vi "Mono Test App.vi"() -> ()   [LabVIEW 2009]
panel:
  in  "BtnCurrent Grating":bool
  out "Current Grating":dbl
  in  "Grating Index":i32
  out "Grating array":dbl[](array[numeric])
  in  "Available Gratings":bool
  in  "Turret Control":bool
  in  "Actual Wavlength":dbl caption="Enter Actual Wavlength"
  in  "Calibrate":bool
  out "Current WL":dbl
  in  "Target WL":dbl
  in  "Get Cur WL":bool
  in  "Move to WL":bool
  in  "Mirror Position  2":u16(ring) caption="Target Position" items=["Front", "Side"]
  in  "Slit Width External":dbl caption="Target Slit Width"
  in  "Slit External":u16(ring) caption="Slit" items=["Front Entrance", "Side Entrance", "Front Exit", "Side Exit", "First Intermediate", "Second Intermediate"]
  out "Slit Width":dbl caption="Current Slit Width"
  in  "Slit":u16(ring) items=["Front Entrance", "Side Entrance", "Front Exit", "Side Exit", "First Intermediate", "Second Intermediate"]
  in  "Set Slit":bool
  in  "Get Slit":bool
  in  "Mirror Number   2":u16(ring) caption="Mirror Number" items=["Entrance", "Exit"]
  in  "Set Mirror Pos":bool
  in  "Get Mirror Pos":bool
  out "Mirror Position":i32(ring) caption="Current  Position" items=["EntranceMirror", "ExitMirror", "Front", "Side"]
  in  "Mirror Number":u16(ring) items=["Entrance", "Exit"]
  in  "stop":bool
  in  "MonoRefNum":refnum<k7>
  out "Initialized":bool
  in  "Force Init":bool
  in  "UniqueID":string
  in  "error in (no error)":errorcluster
  # "Force Init"
  # "Don't Force"
  # "Indexes in this array are zero based"
  # "This requires a 1 based index"
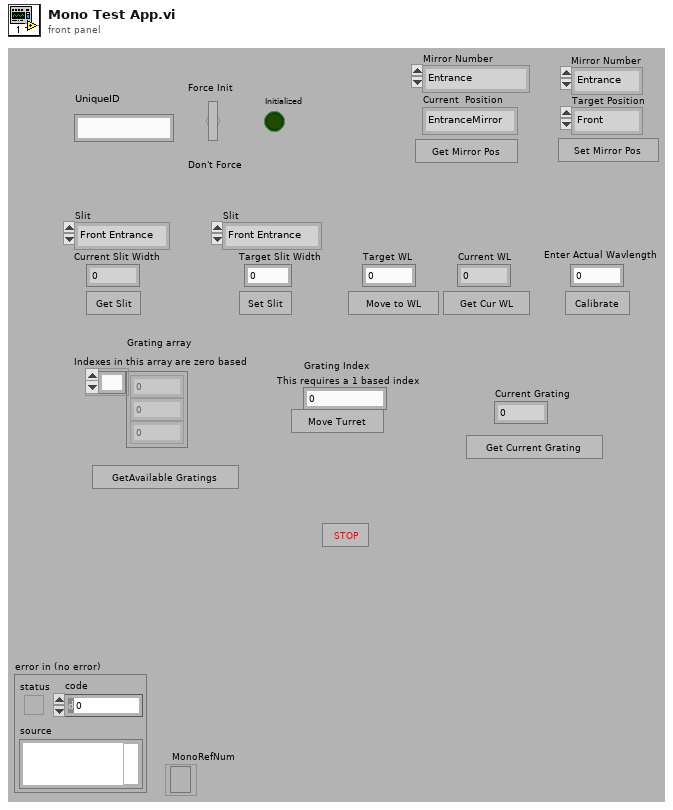
[diagram p1: front panel]
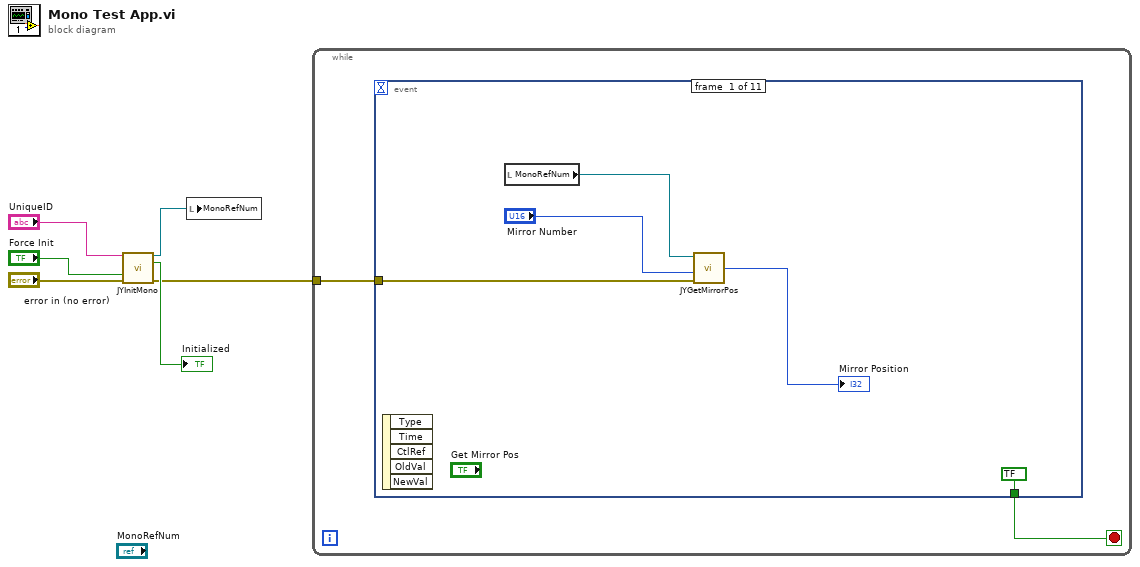
[diagram p0: block diagram]
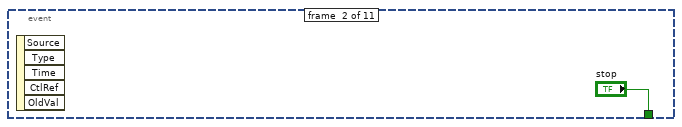
[diagram p2: hidden frame]
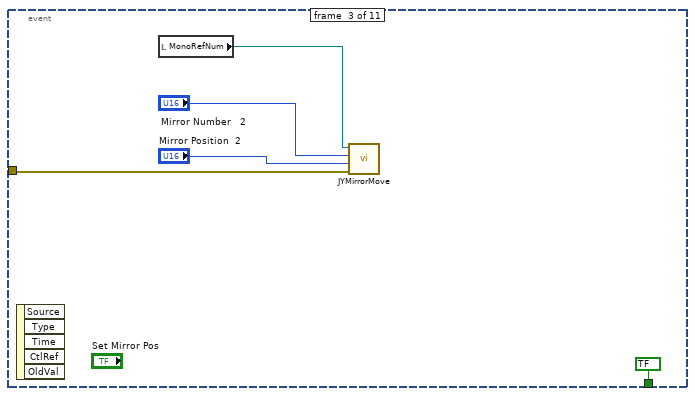
[diagram p3: hidden frame]
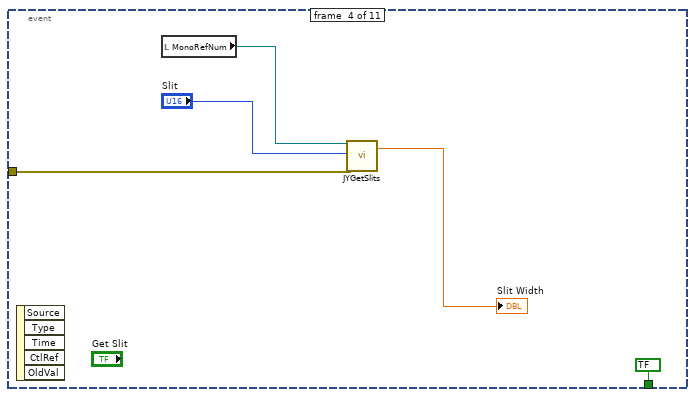
[diagram p4: hidden frame]
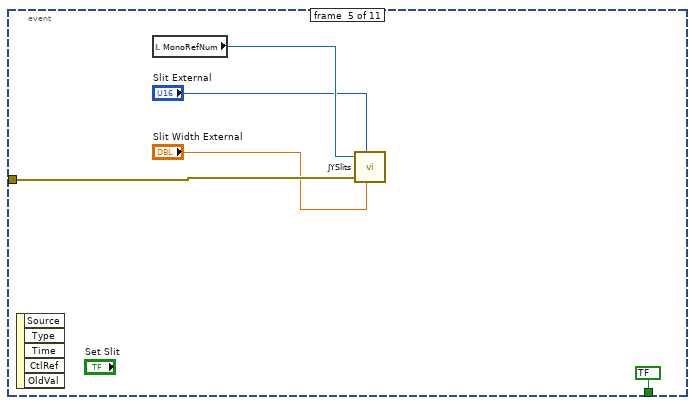
[diagram p5: hidden frame]
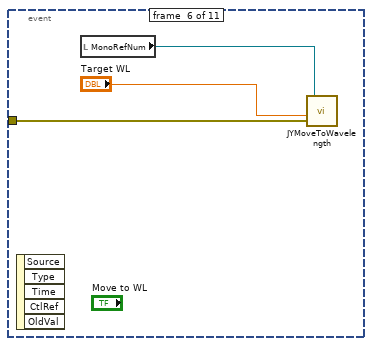
[diagram p6: hidden frame]
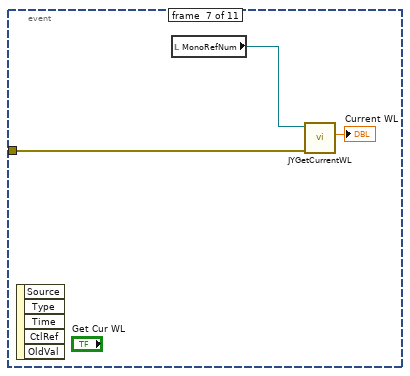
[diagram p7: hidden frame]
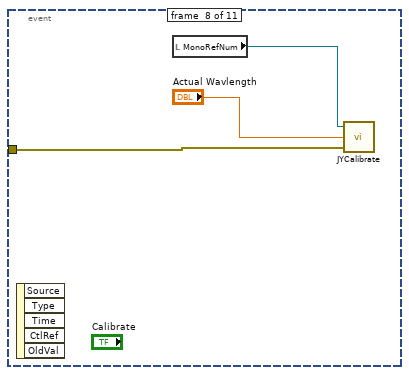
[diagram p8: hidden frame]
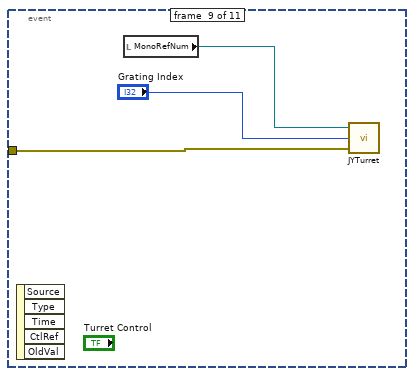
[diagram p9: hidden frame]
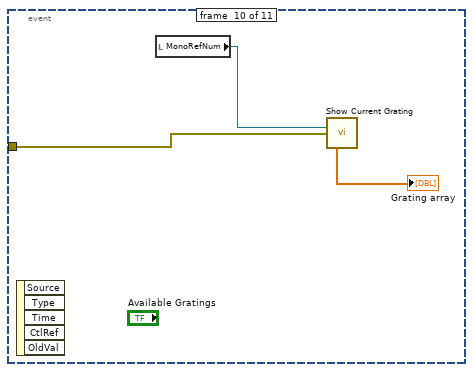
[diagram p10: hidden frame]
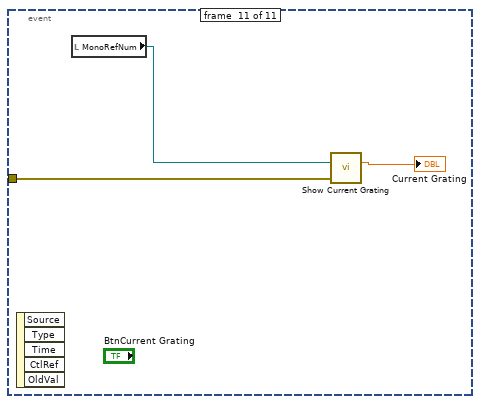
[diagram p11: hidden frame]
diagram:
  n1 = call "JYInitMono.vi"("Unique ID"="UniqueID", "Force Init"="Force Init", "error in (no error)"="error in (no error)") -> ("Mono RefNum out"=w2:refnum<k7>, "Initialized"=→"Initialized":bool, "error out"=w1:errorcluster)  [unwired: 1 in, 9 out]
  n2 = local write "MonoRefNum"(w2) -> ()
  n3 = while {
    tunnel: w1 -> [w8]
    stop <- w7 stop-if-true
    n4 = event shown="[8] \"Turret Control\": Value Change" {
      selector: _ -> [_ _ _ _ _ _ _ _ _ _ _]
      dyn-events: _ -> [_ _ _ _ _ _ _ _ _ _ _]
      timeout: _ -> [_ _ _ _ _ _ _ _ _ _ _]
      tunnel: w8 -> [w10 _ w17 w24 w29 w32 w35 w38 w41 w43 w47]
      tunnel: [bool ? ("stop") "stop" bool ? ("stop") bool ? ("stop") bool ? ("stop") _ _ _ _ _ _] -> w7
      event #0 {
        n5 = event-data() -> ()  [unwired: 6 out]
        n6 = local read "MonoRefNum"() -> (w12:refnum<k7>)
        n7 = call "JYGetMirrorPos.vi"("error in (no error)"=w10, "Mirror"="Mirror Number", "Refnum In"=w12) -> ("Current Mirror Position"=→"Mirror Position":i32)  [unwired: 1 in, 2 out]
      }
      event #1 {
        n8 = event-data() -> ()  [unwired: 6 out]
      }
      event #2 {
        n9 = event-data() -> ()  [unwired: 6 out]
        n10 = local read "MonoRefNum"() -> (w18:refnum<k7>)
        n11 = call "JYMirrorMove.vi"("error in (no error)"=w17, "Mirror Position"="Mirror Position  2", "Mirror Number"="Mirror Number   2", "RefNum In"=w18) -> ()  [unwired: 1 in, 7 out]
      }
      event #3 {
        n12 = event-data() -> ()  [unwired: 6 out]
        n13 = local read "MonoRefNum"() -> (w23:refnum<k7>)
        n14 = call "JYGetSlits.vi"("MonoRefNum IN"=w23, "Slit"="Slit", "error in (no error)"=w24) -> ("Slit Width"=→"Slit Width":dbl)  [unwired: 1 in, 15 out]
      }
      event #4 {
        n15 = event-data() -> ()  [unwired: 6 out]
        n16 = local read "MonoRefNum"() -> (w28:refnum<k7>)
        n17 = call "JYSlits.vi"("JYMONOLib.IJYMonoReqd"=w28, "Slit"="Slit External", "error in (no error)"=w29, "Slit Width"="Slit Width External") -> ()  [unwired: 1 in, 2 out]
      }
      event #5 {
        n18 = event-data() -> ()  [unwired: 6 out]
        n19 = local read "MonoRefNum"() -> (w31:refnum<k7>)
        n20 = call "JYMoveToWavelength.vi"("error in (no error)"=w32, "Target WL"="Target WL", "RefNum In"=w31) -> ()  [unwired: 1 in, 3 out]
      }
      event #6 {
        n21 = event-data() -> ()  [unwired: 6 out]
        n22 = local read "MonoRefNum"() -> (w34:refnum<k7>)
        n23 = call "JYGetCurrentWL.vi"("error in (no error)"=w35, "JYMONOLib.IJYMonoReqd"=w34) -> ("Current WL"=→"Current WL":dbl)  [unwired: 1 in, 8 out]
      }
      event #7 {
        n24 = event-data() -> ()  [unwired: 6 out]
        n25 = local read "MonoRefNum"() -> (w36:refnum<k7>)
        n26 = call "JYCalibrate.vi"("error in (no error)"=w38, "Actual Wavelength"="Actual Wavlength", "JYMONOLib.IJYMonoReqd"=w36) -> ()  [unwired: 2 out]
      }
      event #8 {
        n27 = event-data() -> ()  [unwired: 6 out]
        n28 = local read "MonoRefNum"() -> (w40:refnum<k7>)
        n29 = call "JYTurret.vi"("error in (no error)"=w41, "Grating Index"="Grating Index", "JYMONOLib.IJYMonoReqd"=w40) -> ()  [unwired: 3 out]
      }
      event #9 {
        n30 = event-data() -> ()  [unwired: 6 out]
        n31 = local read "MonoRefNum"() -> (w44:refnum<k7>)
        n32 = call "Show Current Grating.vi"("Refnum in"=w44, "error in (no error)"=w43) -> ("Gratings"=→"Grating array":dbl[])  [unwired: 1 in, 12 out]
      }
      event #10 {
        n33 = event-data() -> ()  [unwired: 6 out]
        n34 = local read "MonoRefNum"() -> (w46:refnum<k7>)
        n35 = call "Show Current Grating.vi"("Refnum in"=w46, "error in (no error)"=w47) -> ("Current Grating"=→"Current Grating":dbl)  [unwired: 1 in, 12 out]
      }
    }
  }
